vi "Is status ongoing - enum.vi"(1 "Monkey Status":T1=enum."Ongoing") -> (0 "Monkey Running?":bool)   [LabVIEW 2020, in "TALOS.lvlib" / "Tamer.lvlib" / "Tamer.lvclass"]
uses:
  Tamer.lvclass
  Run Utilities/TypeDefs/Monkey Status.ctl
  Run Utilities/Run Utilities.lvlib
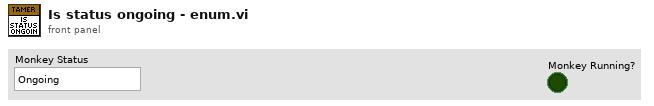
[diagram p1: front panel]
types:
  T1 = typedef "TALOS.lvlib/Run Utilities.lvlib/Monkey Status.ctl" = enum16{"Init", "Paused", "Ongoing", "Stopped", "Finished (no errors)", "Finished (with errors)"}
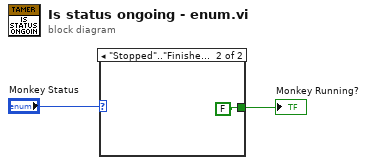
[diagram p0: block diagram]
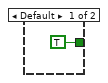
[diagram p2: hidden frame]
diagram:
  n1 = case shown="\"Stopped\"..\"Finished (with errors)\"" "Monkey Status" {
    tunnel: [TRUE FALSE] -> w2
    frame Default {
    }
    frame "Stopped".."Finished (with errors)" {
    }
  }
  "Monkey Running?" <- w2
